vi "Sets the ACW HI SET current value for MANU.vi"(5 "Enable to Query":bool, 7 "Enable to Setup":bool, 8 "error in":errorcluster, 10 "ACW HI SET current value(mA)":sgl=42.0 min=0.001 max=42 format="%.3f", 11 "VISA resource name":refnum<visa-resource-name>) -> (0 "error out":errorcluster, 2 "Return the ACW HI SET current value":string, 3 "VISA resource name out":refnum<visa-resource-name>)   [LabVIEW 2011, in "GPT-9000.lvlib"]
uses:
  <instrlib>/GPT-9000/GPT-9000.lvlib
panel:
  # "mA"
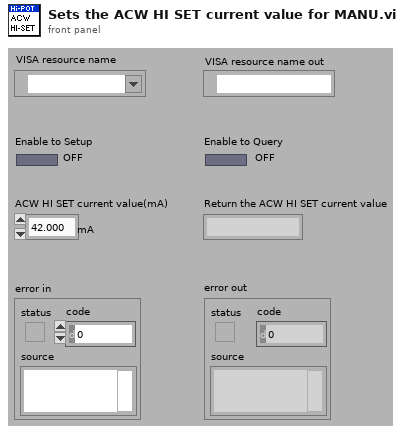
[diagram p1: front panel]
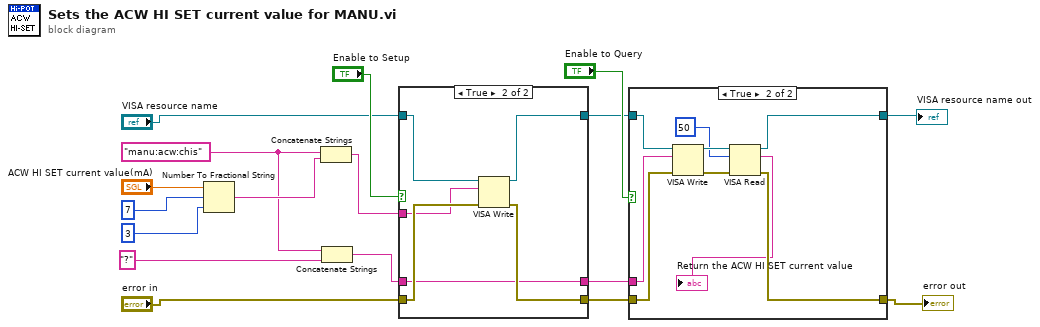
[diagram p0: block diagram]
diagram:
  w12 = "manu:acw:chis"
  n1 = Number To Fractional String(number="ACW HI SET current value(mA)", width (-)=i16 7, precision (6)=i16 3) -> (F-format string=w14:string)  [unwired: 1 in]
  n2 = Concatenate Strings(w12, w14) -> (w10:string)
  n3 = Concatenate Strings(w12, "?") -> (w9:string)
  n4 = case shown="True" "Enable to Setup" {
    tunnel: w10 -> [_ w21]
    tunnel: w9 -> [w18 w22]
    tunnel: "VISA resource name" -> [w20 w26]
    tunnel: "error in" -> [w19 w25]
    tunnel: [w20 w24] -> w5
    tunnel: [w19 w23] -> w4
    tunnel: [w18 w22] -> w3
    frame False {
    }
    frame True {
      n5 = VISA Write(VISA resource name=w26, write buffer=w21, error in (no error)=w25) -> (VISA resource name out=w24:refnum<visa-resource-name>, error out=w23:errorcluster)  [unwired: 1 out]
    }
  }
  n6 = case shown="True" "Enable to Query" {
    tunnel: w5 -> [w28 w36]
    tunnel: w4 -> [w27 w35]
    tunnel: w3 -> [_ w37]
    tunnel: [w28 w31] -> w2
    tunnel: [w27 w30] -> w1
    frame False {
    }
    frame True {
      n7 = VISA Write(VISA resource name=w36, write buffer=w37, error in (no error)=w35) -> (VISA resource name out=w33:refnum<visa-resource-name>, error out=w34:errorcluster)  [unwired: 1 out]
      n8 = VISA Read(VISA resource name=w33, byte count=u32 50, error in (no error)=w34) -> (VISA resource name out=w31:refnum<visa-resource-name>, read buffer=→"Return the ACW HI SET current value":string, error out=w30:errorcluster)  [unwired: 1 out]
    }
  }
  "VISA resource name out" <- w2
  "error out" <- w1
